vi "Update legend.vi"(0 "XYGraph in":refnum<vi>, 5 "max rows":i32, 7 "Listbox":refnum<vi>, 11 "error in (no error)":errorcluster) -> (15 "error out":errorcluster)   [LabVIEW 2020, in "KLegend.xctl"]
uses:
  KLegend.xctl
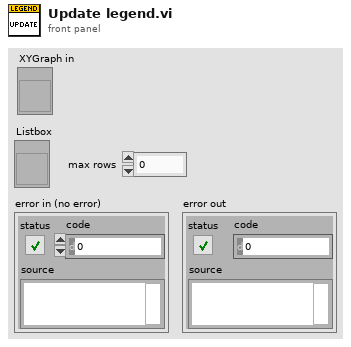
[diagram p1: front panel]
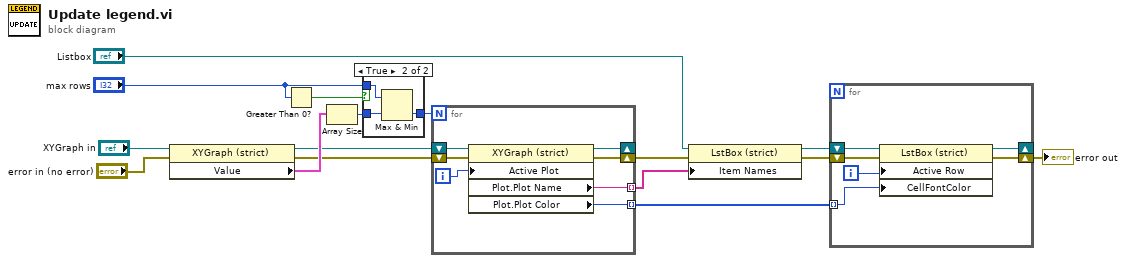
[diagram p0: block diagram]
diagram:
  n1 = property class="XYGraph (strict)"(reference="XYGraph in", error in="error in (no error)") -> (reference out=w13:refnum<vi>, error out=w12:errorcluster, "Value"=w14:cluster{"I-O Plot":dbl[], "I-O Plot":dbl[]}[])
  n2 = Greater Than 0?(x="max rows") -> (x > 0?=w1:bool)
  n3 = Array Size(array=w14) -> (size(s)=w4:i32)
  n4 = case shown="True" w1 {
    tunnel: w4 -> [w17 w20]
    tunnel: [w17 w19] -> w3
    tunnel: "max rows" -> [_ w18]
    frame False {
    }
    frame True {
      n5 = Max & Min(x=w18, y=w20) -> (min(x,y)=w19:i32)  [unwired: 1 out]
    }
  }
  n6 = for {
    N: w3 -> [_]
    shift-right: [w23] -> w10
    shift-left: w12 -> [w27]
    shift-right: [w22] -> _
    shift-left: w13 -> [w26]
    tunnel: [w24] -> w9 mode=indexing
    tunnel: [w21] -> w6 mode=indexing
    i -> [w25]
    n7 = property class="XYGraph (strict)"(reference=w26, error in=w27, "Active Plot"=w25) -> (reference out=w22:refnum<vi>, error out=w23:errorcluster, "Plot.Plot Name"=w24:string, "Plot.Plot Color"=w21:u32)
  }
  n8 = property class="LstBox (strict)"(reference="Listbox", error in=w10, "Item Names"=w9) -> (reference out=w8:refnum<vi>, error out=w7:errorcluster)
  n9 = for {
    shift-right: [w29] -> w5
    shift-left: w7 -> [w32]
    shift-right: [w28] -> _
    shift-left: w8 -> [w33]
    tunnel: w6 -> [w30] mode=indexing
    i -> [w31]
    n10 = property class="LstBox (strict)"(reference=w33, error in=w32, "Active Row"=w31, "CellFontColor"=w30) -> (reference out=w28:refnum<vi>, error out=w29:errorcluster)
  }
  "error out" <- w5
